vi "Send Trigger.vi"(8 "error in":errorcluster, 11 "3300 in":refnum<class "3300.lvclass">) -> (0 "error out":errorcluster, 2 "Snapshot_Data":waveform(dbl)[](array[waveform]), 3 "3300 out":refnum<class "3300.lvclass">)   [LabVIEW 2019, in "3300.lvlib" / "3300.lvclass"]
uses:
  Library/3300.lvclass
  Library/3300.lvclass/3300.ctl
  <instrlib>/Agilent N330X Series/Agilent N330X Series.lvlib
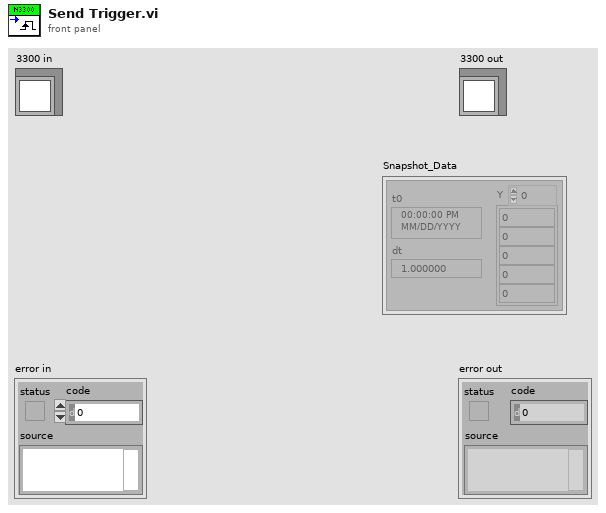
[diagram p1: front panel]
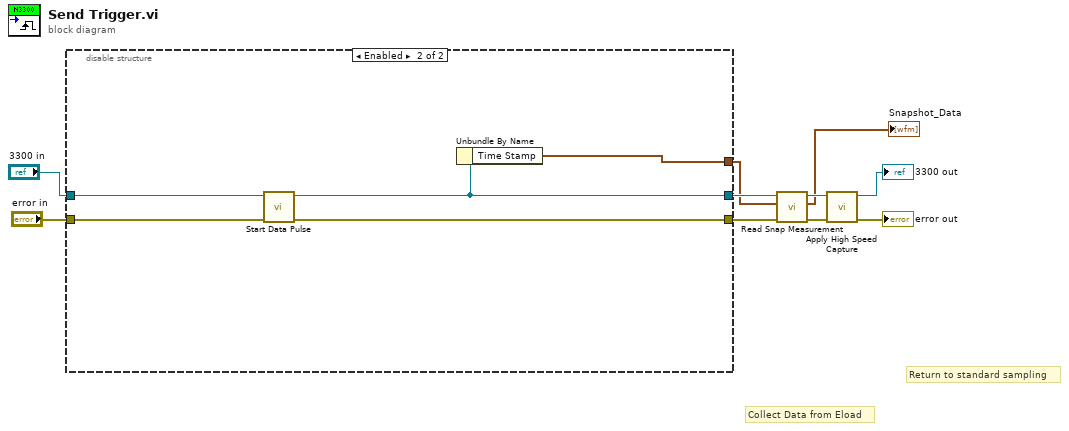
[diagram p0: block diagram]
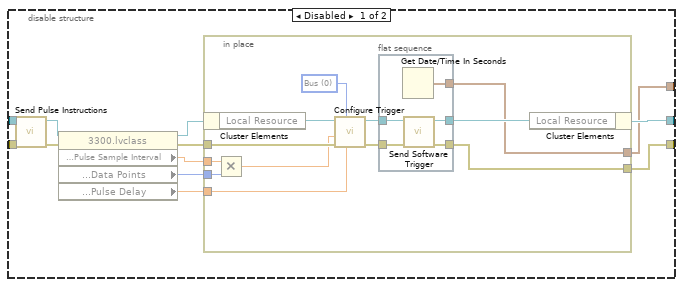
[diagram p2: hidden frame]
diagram:
  # "Collect Data from Eload"
  # "Return to standard sampling"
  n1 = disable-structure shown="Enabled" {
    disable-tunnel: "3300 in" -> [w22 w44]
    disable-tunnel: "error in" -> [w21 w43]
    disable-tunnel: [w20 w42] -> w3
    disable-tunnel: [w19 w41] -> w2
    disable-tunnel: [w11 w40] -> w1
    frame Disabled {
      n2 = call "Send Pulse Instructions.vi"("error in"=w21, "3300 in"=w22) -> ("error out"=w16:errorcluster, "3300 out"=w18:refnum<class "3300.lvclass">)  [unwired: 8 in]
      n3 = property class="3300.lvclass"(reference=w18, error in=w16) -> (reference out=w17:refnum<class "3300.lvclass">, error out=w15:errorcluster, "Accessors:Settings:Pulse:Pulse Sample Interval"=w12:dbl, "Accessors:Settings:Pulse:Data Points"=w13:i32, "Accessors:Settings:Pulse:Pulse Delay"=w14:dbl)
      n4 = in-place {
        in-place-border: w15 -> [w30]
        in-place-border: [w28] -> w20
        in-place-border: [w27] -> w11
        in-place-border: w14 -> [w26]
        in-place-border: w13 -> [w25]
        in-place-border: w12 -> [w24]
        w32 = 0 items=["Bus", "External", "Hold", "Line", "Timer"] ("Trigger Source (2: Hold)")
        n5 = in-place-cluster #1(w17) -> ("Local Resource"=w31:refnum<visa-resource-name>)
        n6 = Multiply(x=w24, y=w25) -> (x*y=w23:dbl)
        n7 = call <instrlib>:"Configure Trigger.vi"("Trigger Delay (0 s)"=w26, "Trigger Source (2: Hold)"=w32, "error in (no error)"=w30, "Trigger Period (0.001 s)"=w23, "VISA resource name"=w31) -> ("error out"=w33:errorcluster, "VISA resource name out"=w34:refnum<visa-resource-name>)  [unwired: 5 in]
        n8 = flat-sequence {
          tunnel: w34 -> [w39]
          tunnel: w33 -> [w38]
          tunnel: [w37] -> w29
          tunnel: [w36] -> w28
          tunnel: [w35] -> w27
          frame #0 {
            n9 = Get Date/Time In Seconds() -> (seconds since 1Jan1904=w35:timestamp)
            n10 = call <instrlib>:"Send Software Trigger.vi"("error in (no error)"=w38, "VISA resource name"=w39) -> ("error out"=w36:errorcluster, "VISA resource name out"=w37:refnum<visa-resource-name>)  [unwired: 8 in]
          }
        }
        n11 = in-place-cluster #1("Local Resource"=w29) -> (w19:refnum<class "3300.lvclass">)
      }
    }
    frame Enabled {
      n12 = call-dynamic "Start Data Pulse.vi"("error in (no error)"=w43, "3300 in"=w44) -> ("error out"=w42:errorcluster, "3300 out"=w41:refnum<class "3300.lvclass">)  [unwired: 8 in]
      n13 = Unbundle By Name(w41) -> ("Time Stamp"=w40:timestamp)
    }
  }
  n14 = call "Read Snap Measurement.vi"("error in"=w3, "Trigger_Start"=w1, "3300 in"=w2) -> ("error out"=w7:errorcluster, "Snapshot Data"=→"Snapshot_Data":waveform(dbl)[], "3300 out"=w8:refnum<class "3300.lvclass">)  [unwired: 6 in]
  n15 = call "Apply High Speed Capture.vi"("error in"=w7, "3300 in"=w8) -> ("error out"=→"error out":errorcluster, "3300 out"=→"3300 out":refnum<class "3300.lvclass">)  [unwired: 8 in]
